vi "File.Write.vi"(8 "error in":errorcluster, 9 "pos mode (end)":enum16{"start", "end", "current"}(ring)=enum."end", 10 "Text":string, 11 "File ref in":refnum<file>) -> (0 "error out":errorcluster, 3 "File ref out":refnum<file>)   [LabVIEW 2015]
doc: "Writes to a file.\nIf <B>append</B> is false (default), the file will be rewritten.\nIf <B>append</B> is true, the new data will be appended to the file.\nSupports a <B>header</B> line which will be placed on top of the file when it is created or rewritten. This <B>header</B> line requires a newline at the end."
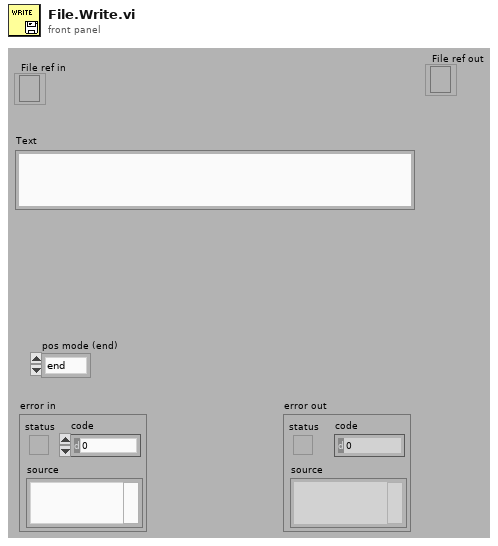
[diagram p1: front panel]
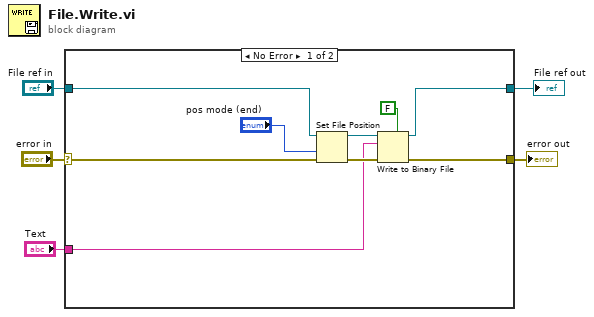
[diagram p0: block diagram]
diagram:
  n1 = case shown="No Error" "error in" {
    selector: "error in" -> [w9 w16]
    tunnel: [w14 w16] -> w5
    tunnel: "Text" -> [w10 _]
    tunnel: "File ref in" -> [w8 w15]
    tunnel: [w7 w15] -> w1
    frame No Error {
      n2 = Set File Position(refnum=w8, from (0:start)="pos mode (end)", error in=w9) -> (refnum out=w13:refnum<file>, error out=w12:errorcluster)  [unwired: 1 out]
      n3 = Write to Binary File(file (use dialog)=w13, data=w10, error in=w12, 5:FALSE ("prepend array or string size? (T)")) -> (refnum out=w7:refnum<file>, error out=w14:errorcluster)  [unwired: 3 out]
    }
    frame Error {
    }
  }
  "error out" <- w5
  "File ref out" <- w1
